vi "PKG_IMC_AxisMap.vi"(7 "fifo":i32, 9 "num":i32, 10 "axis":i32[](array[numeric])=array[4097 elements], 11 "handle":u32) -> (1 "function return":i32, 2 "axis out":i32[](array[numeric]), 3 "handle out":u32)   [LabVIEW 2011, in "IMC_Pkg4xxx.lvlib"]
doc: "PKG_IMC_AxisMap(IMC_HANDLE handle, int axis[], int num, int fifo);"
uses:
  IMC_Pkg4xxx.lvlib
  IMC_Pkg4xxx.dll
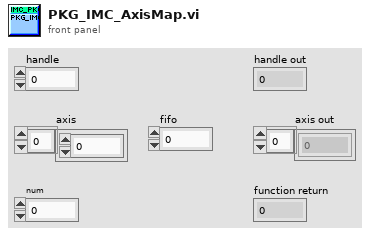
[diagram p1: front panel]
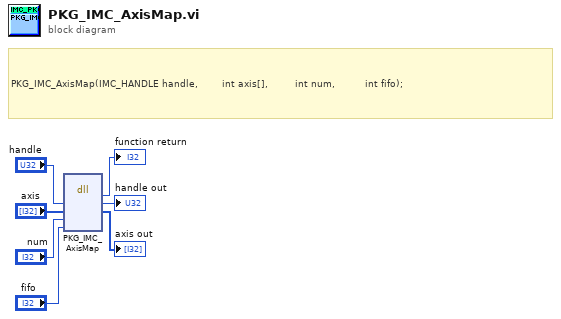
[diagram p0: block diagram]
diagram:
  # "PKG_IMC_AxisMap(IMC_HANDLE handle, \t\t\t\t\t\t\tint axis[], \t\t\t\t\t\t\t\tint num, \t\t\t\t\t\t\t\t\tint fifo);"
  n1 = dll-call lib="PTH1mabs F光盘刻录\niMC MotionIMCNet_V4.0IMCAppincLabviewIMC_PKG4xxxIMC_PKG4xxx\nIMC_Pkg4xxx.*" fn="PKG_IMC_AxisMap"("handle"="handle", "axis"="axis", "num"="num", "fifo"="fifo") -> (→"function return":i32, "handle"=→"handle out":u32, "axis"=→"axis out":i32[])  [unwired: 5 in, 2 out]
